vi "默认配置-多点监测.vi"(11 "配置内容（结构）":T1={"COM"="", "探头地址"=[], "探头启用状态？"=[], "开机启动？"=FALSE, "探头信息"=[], "限值"=[], "最大探头数"=0, "波特率"=enum."19200", "周期"=0, "报警方式"=[], "静音延迟"=0}) -> (3 "默认配置":T2={"COM"="", "探头地址"=[], "探头启用状态？"=[], "开机启动？"=FALSE, "探头信息"=[], "限值"=[], "最大探头数"=0, "波特率"=enum."19200", "周期"=3600000, "初始化的数组"=[], "静音延迟"=0})   [LabVIEW 2017]
uses:
  <vilib>/Instr/_visa.llb/VISA Find Search Mode.ctl
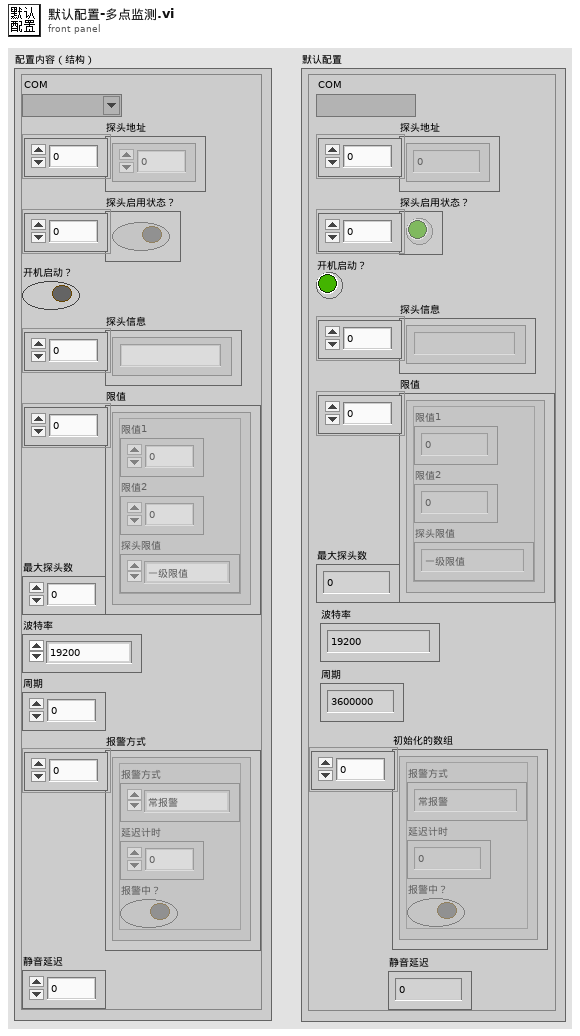
[diagram p1: front panel]
types:
  T1 = cluster{"COM":refnum<visa-resource-name>, "探头地址":i32[], "探头启用状态？":bool[], "开机启动？":bool, "探头信息":string[], "限值":cluster{"限值1":dbl, "限值2":dbl, "探头限值":enum16{"一级限值", "二级限值"}}[], "最大探头数":i32, "波特率":enum16{"9600", "19200"}, "周期":i64, "报警方式":cluster{"报警方式":enum16{"常报警", "自动静音", "手动静音"}, "延迟计时":u16, "报警中？":bool}[], "静音延迟":u16}
  T2 = cluster{"COM":refnum<visa-resource-name>, "探头地址":i32[], "探头启用状态？":bool[], "开机启动？":bool, "探头信息":string[], "限值":cluster{"限值1":dbl, "限值2":dbl, "探头限值":enum16{"一级限值", "二级限值"}}[], "最大探头数":i32, "波特率":enum16{"9600", "19200"}, "周期":i64, "初始化的数组":cluster{"报警方式":enum16{"常报警", "自动静音", "手动静音"}, "延迟计时":u16, "报警中？":bool}[], "静音延迟":u16}
  T3 = cluster{"限值1":dbl, "限值2":dbl, "探头限值":enum16{"一级限值", "二级限值"}}
  T4 = cluster{"报警方式":enum16{"常报警", "自动静音", "手动静音"}, "延迟计时":u16, "报警中？":bool}
  T5 = typedef "VISA Find Search Mode.ctl" = u32
  T6 = cluster{"限值1":dbl, "限值2":dbl, "探头限值":enum16{"一级限值", "二级限值"}}[]
  T7 = cluster{"报警方式":enum16{"常报警", "自动静音", "手动静音"}, "延迟计时":u16, "报警中？":bool}[]
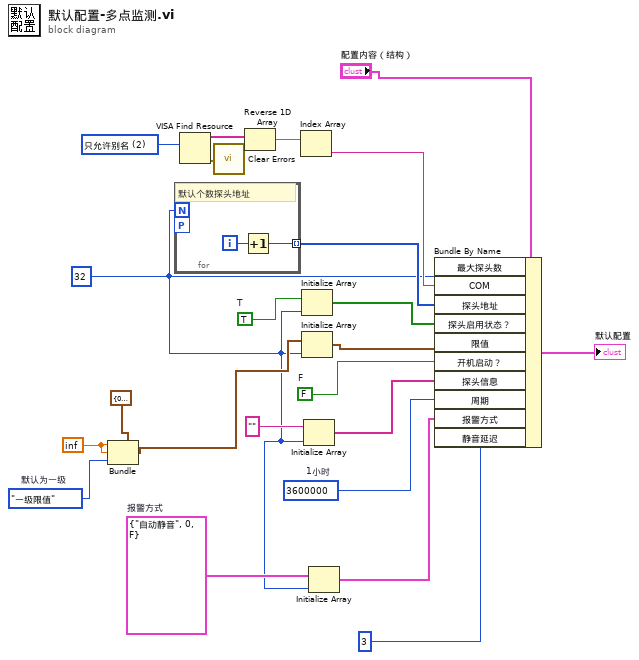
[diagram p0: block diagram]
diagram:
  w1 = enum16{"一级限值", "二级限值"}."一级限值"  # 默认为一级
  w7 = T4 {"报警方式"=enum."自动静音", "延迟计时"=0, "报警中？"=FALSE}  # 报警方式
  w8 = i64 3600000  # 1小时
  w11 = inf
  w6 = 32 ("最大探头数")
  w17 = FALSE  # F
  w23 = T5 2 items=["仅允许规范名称"=0, "只允许别名"=2, "包含匹配别名"=3, "包含所有别名"=4] ("Search Mode")
  w19 = TRUE  # T
  n1 = Bundle(cluster=T3 {"限值1"=0.0, "限值2"=0.0, "探头限值"=enum."一级限值"} ("探头限值簇"), "限值1"=w11, "限值2"=w11, "探头限值"=w1) -> (w10:T3)
  n2 = for {
    N: w6 -> [_]
    workers-P: _ -> [_]
    tunnel: [w24] -> w20 mode=indexing
    i -> [w25]
    # "默认个数探头地址"
    n3 = Increment(x=w25) -> (x+1=w24:i32)
  }
  n4 = VISA Find Resource(10:w23) -> (0:w9:errorcluster, 3:w22:string[])  [unwired: 2 in, 1 out]
  n5 = call <vilib>:"Clear Errors.vi"("error in (no error)"=w9) -> ()  [unwired: 5 in, 2 out]
  n6 = Reverse 1D Array(array=w22) -> (reversed array=w15:string[])
  n7 = Index Array(array=w15) -> (element=w21:string)  [unwired: 1 in]
  n8 = Initialize Array(w19, w6) -> (w18:bool[])
  n9 = Initialize Array(w10, w6) -> (w13:T6)
  n10 = Initialize Array("", w6) -> (w14:string[])
  n11 = Initialize Array(w7, w6) -> (w5:T7)
  n12 = Bundle By Name(cluster="配置内容（结构）", "最大探头数"=w6, "COM"=w21, "探头地址"=w20, "探头启用状态？"=w18, "限值"=w13, "开机启动？"=w17, "探头信息"=w14, "周期"=w8, "报警方式"=w5, "静音延迟"=u16 3) -> (→"默认配置":T1)
